vi "Build Async Payload.vi"(8 "error in (no error)":errorcluster, 10 "Async Pointers":T2 {"LP Async Data Addresses" format="%04x"; "LP Async Control Addresses" format="%04x"; "HP Async Data Addresses" format="%04x"; "HP Async Control Addresses" format="%04x"}, 11 "Async RT-RT Message in":refnum<class "Async RT-RT Message.lvclass">) -> (0 "error out":errorcluster, 2 "Async Payload":T1 {"Trigger Command" format="%04x"; "Data" format="%04x"; "Data Address" format="%04x"; "Configuration" format="%04x"; "Configuration Address" format="%04x"}, 3 "Async RT-RT Message out":refnum<class "Async RT-RT Message.lvclass">)   [LabVIEW 2020, in "BCI-1553 API.lvlib" / "Async RT-RT Message.lvclass"]
doc: "Builds the data payload that will need to be sent down to the Holt IC by the caller."
uses:
  Async RT-RT Message.lvclass
  TypeDefs/Async Message Pointers.ctl
  TypeDefs/Async Payload.ctl
  BCI-1553 API.lvlib
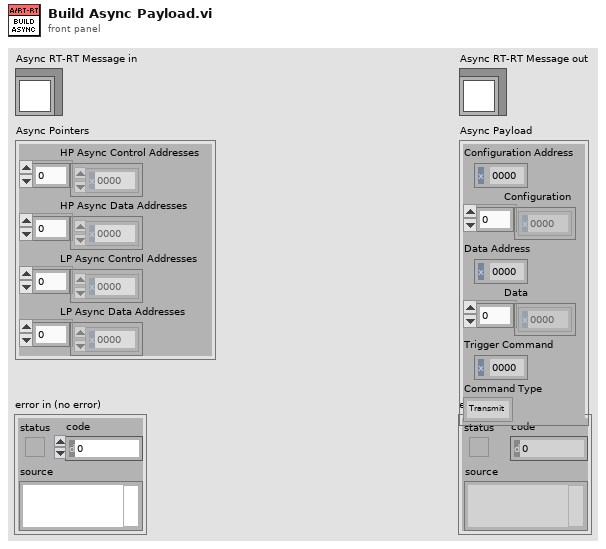
[diagram p1: front panel]
types:
  T1 = typedef "BCI-1553 API.lvlib/Async Payload.ctl" = cluster{"Configuration Address":u16, "Configuration":u16[], "Data Address":u16, "Data":u16[], "Trigger Command":u16, "Command Type":enum16{"Transmit", "Receive"}}
  T2 = typedef "BCI-1553 API.lvlib/Async Message Pointers.ctl" = cluster{"HP Async Control Addresses":u16[], "HP Async Data Addresses":u16[], "LP Async Control Addresses":u16[], "LP Async Data Addresses":u16[]}
  T3 = typedef "BCI-1553 API.lvlib/Async Message Config.ctl" = cluster{"Group":i32, "High Priority":bool, "Time to Next Msg (100 us)":u16, "Command Config":T4, "Message Control":T9}
  T4 = typedef "BCI-1553 API.lvlib/Command Config.ctl" = cluster{"Command Type":T5, "Terminal Address":T6, "SubAddress":T7, "Word Count\\Mode Code":T8, "Command Data":u16[]}
  T5 = typedef "BCI-1553 API.lvlib/Command Type.ctl" = enum16{"Transmit", "Receive"}
  T6 = typedef "BCI-1553 API.lvlib/Command Terminal Address.ctl" = enum16{"0", "1", "2", "3", "4", "5", "6", "7", "8", "9", "10", "11", "12", "13", "14", "15", "16", "17", "18", "19", "20", "21", "22", "23", "24", "25", "26", "27", "28", "29", "30", "Broadcast"}
  T7 = typedef "BCI-1553 API.lvlib/Command SubAddress.ctl" = enum16{"Mode Code", "1", "2", "3", "4", "5", "6", "7", "8", "9", "10", "11", "12", "13", "14", "15", "16", "17", "18", "19", "20", "21", "22", "23", "24", "25", "26", "27", "28", "29", "30"}
  T8 = typedef "BCI-1553 API.lvlib/Command Word Count.ctl" = enum16{"1", "2", "3", "4", "5", "6", "7", "8", "9", "10", "11", "12", "13", "14", "15", "16", "17", "18", "19", "20", "21", "22", "23", "24", "25", "26", "27", "28", "29", "30", "31", "32"}
  T9 = typedef "BCI-1553 API.lvlib/Message Control.ctl" = cluster{"MC17 Time Sync":bool, "Error Mask":bool, "Service Request Mask":bool, "Busy Mask":bool, "SubSystem Flag Mask":bool, "Terminal Flag Mask":bool, "Reserved Mask":bool, "Retry":bool, "Bus A / !Bus B":bool, "Self-Test Loopback":bool, "Broadcast Mask":bool, "EoM Interrupt":bool, "Mode Code Format":bool, "Broadcast Format":bool, "RT-RT Format":bool}
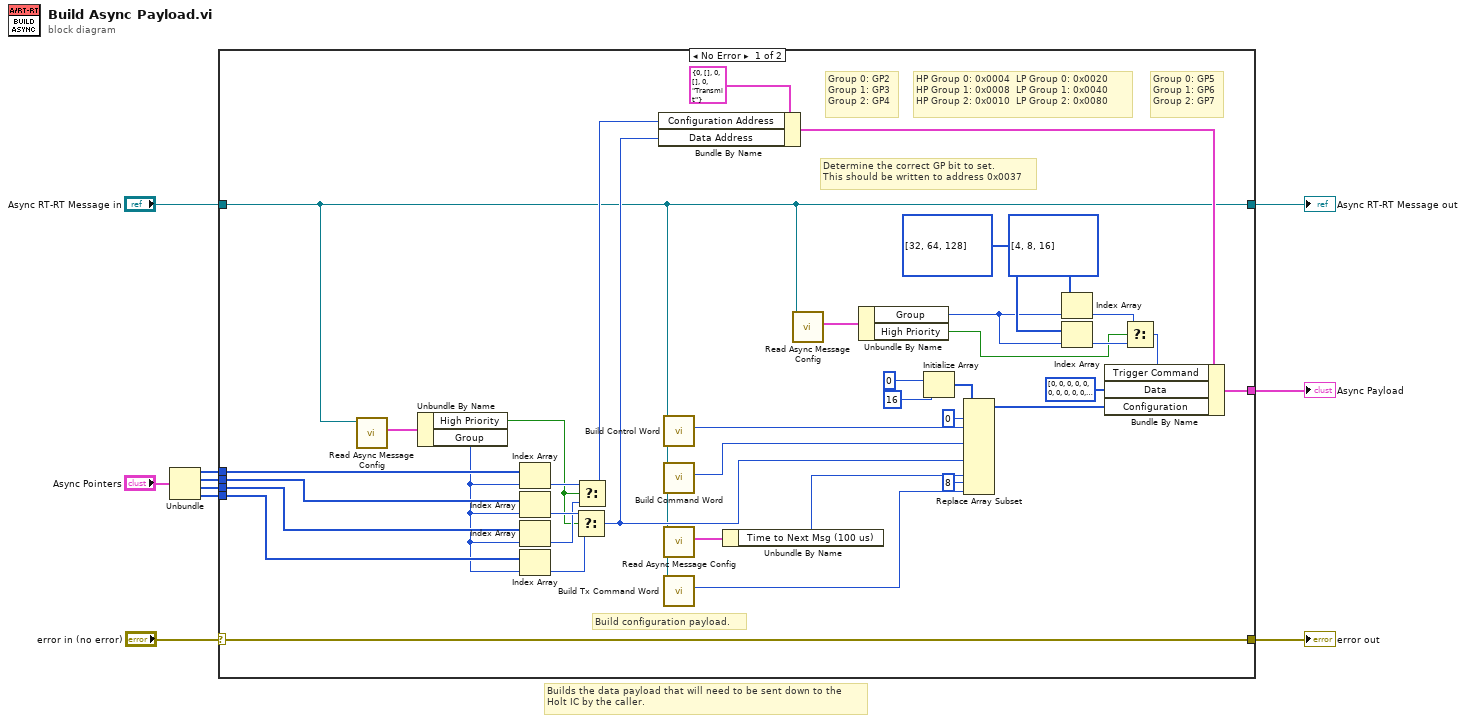
[diagram p0: block diagram]
diagram:
  # "Builds the data payload that will need to be sent down to the\nHolt IC by the caller."
  n1 = Unbundle("Async Pointers") -> ("HP Async Control Addresses"=w8:u16[], "HP Async Data Addresses"=w10:u16[], "LP Async Control Addresses"=w7:u16[], "LP Async Data Addresses"=w9:u16[])
  n2 = case shown="No Error" "error in (no error)" {
    selector: "error in (no error)" -> [w48 w50]
    tunnel: [w48 w50] -> w1
    tunnel: [w13 w49] -> w3
    tunnel: "Async RT-RT Message in" -> [w13 w49]
    tunnel: w10 -> [w46 _]
    tunnel: w9 -> [w47 _]
    tunnel: w8 -> [w35 _]
    tunnel: w7 -> [w36 _]
    tunnel: [w28 _] -> w2
    frame No Error {
      # "Group 0: GP5\nGroup 1: GP6\nGroup 2: GP7"
      # "Group 0: GP2\nGroup 1: GP3\nGroup 2: GP4"
      # "HP Group 0: 0x0004  LP Group 0: 0x0020  \nHP Group 1: 0x0008  LP Group 1: 0x0040  \nHP Group 2: 0x0010  LP Group 2: 0x0080"
      # "Determine the correct GP bit to set.\nThis should be written to address 0x0037"
      # "Build configuration payload."
      n3 = call-dynamic "Read Async Message Config.vi"("Async Message in"=w13) -> ("Async Message Config"=w22:T3)  [unwired: 8 in, 2 out]
      n4 = Unbundle By Name(w22) -> ("High Priority"=w20:bool, "Group"=w21:i32)
      n5 = Index Array(array=w35, index=w21) -> (element=w34:u16)
      n6 = Index Array(array=w46, index=w21) -> (element=w45:u16)
      n7 = Index Array(array=w36, index=w21) -> (element=w33:u16)
      n8 = Index Array(array=w47, index=w21) -> (element=w44:u16)
      n9 = Select(t=w45, s=w20, f=w44) -> (s? t:f=w31:u16)
      n10 = Select(t=w34, s=w20, f=w33) -> (s? t:f=w32:u16)
      n11 = Bundle By Name(cluster=T1 {"Configuration Address"=0, "Configuration"=[], "Data Address"=0, "Data"=[], "Trigger Command"=0, "Command Type"=enum."Transmit"} ("Async Payload"), "Configuration Address"=w32, "Data Address"=w31) -> (w30:T1)
      n12 = call-dynamic "Build Control Word.vi"("Async Message in"=w13) -> ("Control Word"=w39:u16)  [unwired: 9 in, 1 out]
      n13 = call-dynamic "Build Command Word.vi"("Async Message in"=w13) -> ("Command Word"=w38:u16)  [unwired: 9 in, 1 out]
      n14 = call-dynamic "Read Async Message Config.vi"("Async Message in"=w13) -> ("Async Message Config"=w19:T3)  [unwired: 8 in, 2 out]
      n15 = call "Build Tx Command Word.vi"("Async RT-RT Message in"=w13) -> ("Tx Command Word"=w12:u16)  [unwired: 9 in, 1 out]
      n16 = Unbundle By Name(w19) -> ("Time to Next Msg (100 us)"=w18:u16)
      n17 = call-dynamic "Read Async Message Config.vi"("Async Message in"=w13) -> ("Async Message Config"=w17:T3)  [unwired: 8 in, 2 out]
      n18 = Unbundle By Name(w17) -> ("Group"=w15:i32, "High Priority"=w16:bool)
      n19 = Initialize Array(u16 0 ("Command Word"), 16 ("dimension size")) -> (w41:u16[])
      n20 = Replace Array Subset(array=w41, new element #1=w39, index #1=0 ("index"), new element #2=w38, new element #3=w31, new element #4=w18, new element #5=w12, index #5=8 ("index")) -> (w29:u16[])  [unwired: 3 in]
      n21 = Index Array(array=u16[] [4, 8, 16] ("Command Word"), index=w15) -> (element=w25:u16)
      n22 = Index Array(array=u16[] [32, 64, 128] ("Command Word"), index=w15) -> (element=w24:u16)
      n23 = Select(t=w25, s=w16, f=w24) -> (s? t:f=w23:u16)
      n24 = Bundle By Name(cluster=w30, "Trigger Command"=w23, "Data"=u16[] [0, 0, 0, 0, 0, 0, 0, 0, 0, 0, 0, 0, 0, 0, 0, 0, 0, 0, 0, 0, 0, 0, 0, 0, 0, 0, 0, 0, 0, 0, 0, 0], "Configuration"=w29) -> (w28:T1)
    }
    frame Error {
    }
  }
  "error out" <- w1
  "Async RT-RT Message out" <- w3
  "Async Payload" <- w2
